vi "Peak register (no reset).vi"(11 "Value in":dbl) -> (3 "Registered peak value":dbl)   [LabVIEW 2017]
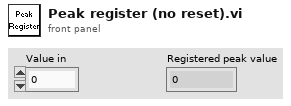
[diagram p1: front panel]
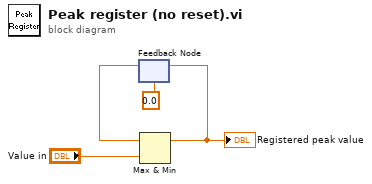
[diagram p0: block diagram]
diagram:
  n1 = feedback #1(0.0) -> (w2:dbl)
  n2 = Max & Min(x=w2, y="Value in") -> (max(x,y)=w3:dbl)  [unwired: 1 out]
  "Registered peak value" <- w3
  n3 = feedback-in #1(w3) -> ()
